vi "libssh2_userauth_keyboard_interactive_ex.vi"(8 "error in (no error)":errorcluster, 10 "username":string, 11 "session":T1) -> (0 "error out":errorcluster)   [LabVIEW 2017, in "libssh2.lvlib"]
doc: "Authenticate a session using keyboard-interactive authentication.\n\nThis function utilizes the lvssh2 extension library. You can disable the extension library by defining the LVSSH2_NO_EXTENSIONS conditional disable symbol with the value 'True' in the project properties. When the extension library is disabled, this function turns into a no-op."
uses:
  libssh2.lvlib
  Session Refnum.ctl
  Not A Session.vi
  <vilib>/Utility/error.llb/Error Cluster From Error Code.vi
  Global Settings.vi
  Read Session Refnum.vi
  <vilib>/Utility/semaphor.llb/Acquire Semaphore.vi
  <vilib>/Utility/semaphor.llb/Release Semaphore.vi
  lvssh2_extensions_64.dll
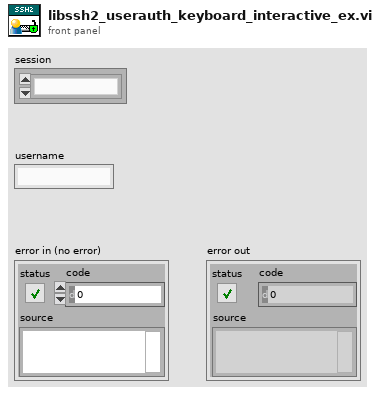
[diagram p1: front panel]
types:
  T1 = typedef "libssh2.lvlib/Session Refnum.ctl" = refnum<k1>
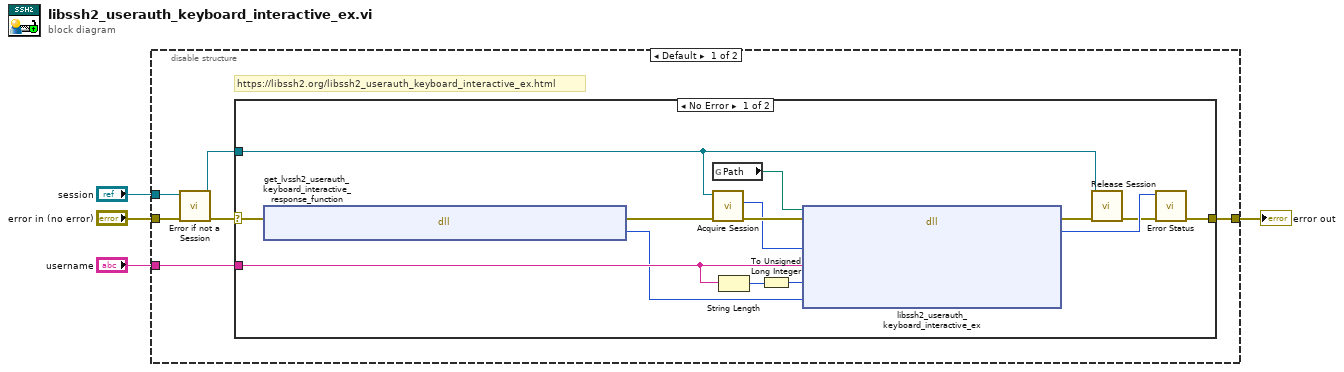
[diagram p0: block diagram]
diagram:
  n1 = disable-structure shown="Default" {
    disable-tunnel: "username" -> [w10 _]
    disable-tunnel: [w9 w26] -> w3
    disable-tunnel: "error in (no error)" -> [w8 w26]
    disable-tunnel: "session" -> [w6 _]
    frame condition #0 (active) {
      # "https://libssh2.org/libssh2_userauth_keyboard_interactive_ex.html"
      n2 = call "Error if not a Session.vi"("error in (no error)"=w8, "session"=w6) -> ("error out"=w7:errorcluster, "session out"=w5:T1)  [unwired: 8 in]
      n3 = case shown="No Error" w7 {
        selector: w7 -> [w14 w25]
        tunnel: w10 -> [w24 _]
        tunnel: [w13 w25] -> w9
        tunnel: w5 -> [w11 _]
        frame No Error {
          n4 = dll-call lib="C:/Users/pasca/Projects/Home/lvssh2/libssh2/lvssh2_extensions**.*" fn="get_lvssh2_userauth_keyboard_interactive_response_function"(error in=w14) -> (error out=w16:errorcluster, "return type"=w15:u64)  [unwired: 2 in, 1 out]
          n5 = global read "Global Settings.vi" "Path"() -> (w18:path)
          n6 = call "Acquire Session.vi"("error in (no error)"=w16, "session"=w11) -> ("error out"=w20:errorcluster, "LIBSSH2_SESSION*"=w19:u64)  [unwired: 7 in, 1 out]
          n7 = String Length(string=w24) -> (length=w21:i32)
          n8 = To Unsigned Long Integer(number=w21) -> (unsigned 32bit integer=w23:u32)
          n9 = dll-call lib="?" fn="libssh2_userauth_keyboard_interactive_ex"(path in=w18, error in=w20, "session"=w19, "username"=w24, "username_len"=w23, "response_callback"=w15) -> (error out=w22:errorcluster, "return value"=w17:i32)  [unwired: 5 in, 1 out]
          n10 = call "Release Session.vi"("error in (no error)"=w22, "session"=w11) -> ("error out"=w12:errorcluster)  [unwired: 9 in]
          n11 = call "Error Status.vi"("error in (no error)"=w12, "return value"=w17) -> ("error out"=w13:errorcluster)  [unwired: 8 in, 1 out]
        }
        frame Error {
        }
      }
    }
    frame condition #1 {
    }
  }
  "error out" <- w3
